vi "Knock Sensor 1.0 Write Inputs.vi"(5 "Device inputs":dbl[](array[numeric]), 6 "DAC multiplier":dbl, 7 "Last Device inputs":dbl[](array[numeric]), 8 "error in (no error)":errorcluster, 9 "input reference in":T1, 10 "input in":cluster{"low freq scaler":fxp<+,10,0>}, 11 "FIFO indexes.inputs":T2) -> (0 "error out":errorcluster, 1 "input reference out":T1, 2 "input out":cluster{"low freq scaler":fxp<+,10,0>})   [LabVIEW 2019, in "Engine Simulation Toolkit Engine.lvlib"]
uses:
  Engine Simulation Toolkit Engine.lvlib
  Shared/1.0 Knock Sensor FIFO Idxs.ctl
  Knock Sensor 1.0 Input Ref.ctl
  Shared/Engine Simulation Toolkit Shared.lvlib
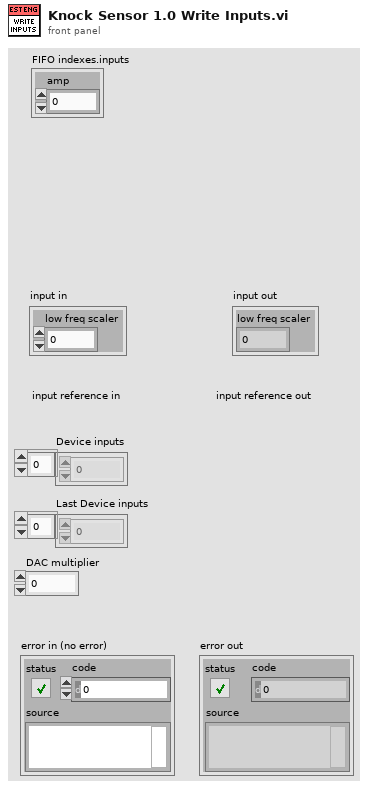
[diagram p1: front panel]
types:
  T1 = typedef "Engine Simulation Toolkit Engine.lvlib/Knock Sensor 1.0 Input Ref.ctl" = refnum<k20>
  T2 = typedef "Engine Simulation Toolkit Shared.lvlib/1.0 Knock Sensor FIFO Idxs.ctl" = cluster{"amp":i32}
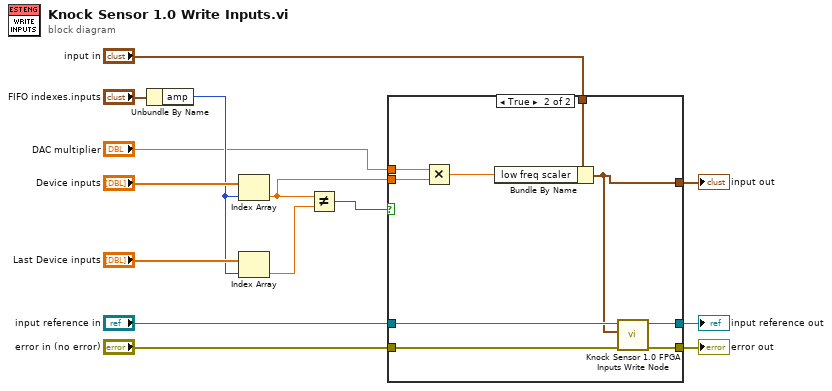
[diagram p0: block diagram]
diagram:
  n1 = Unbundle By Name("FIFO indexes.inputs") -> ("amp"=w7:i32)
  n2 = Index Array(array="Device inputs", index=w7) -> (element=w4:dbl)
  n3 = Index Array(array="Last Device inputs", index=w7) -> (element=w5:dbl)
  n4 = Not Equal?(x=w4, y=w5) -> (x != y?=w2:bool)
  n5 = case shown="True" w2 {
    tunnel: "error in (no error)" -> [w15 w26]
    tunnel: "input reference in" -> [w16 w19]
    tunnel: [w15 w25] -> w12
    tunnel: [w16 w24] -> w1
    tunnel: "input in" -> [w17 w23]
    tunnel: [w17 w18] -> w6
    tunnel: w4 -> [_ w22]
    tunnel: "DAC multiplier" -> [_ w21]
    frame False {
    }
    frame True {
      n6 = Multiply(x=w21, y=w22) -> (x*y=w20:dbl)
      n7 = Bundle By Name(cluster=w23, "low freq scaler"=w20) -> (w18:cluster{"low freq scaler":fxp<+,10,0>})
      n8 = call "Knock Sensor 1.0 FPGA Inputs Write Node.vi"("error in (no error)"=w26, "input"=w18, "Refnum in"=w19) -> ("error out"=w25:errorcluster, "Refnum out"=w24:T1)  [unwired: 7 in]
    }
  }
  "error out" <- w12
  "input out" <- w6
  "input reference out" <- w1
